vi "Add Canvas Wfm To Save.vi"(7 "Canvas Trim and Resample Settings":cluster{"Duration":dbl, "Sample Rate":dbl}={"Duration"=0.002, "Sample Rate"=0.0} {"Sample Rate" format="%#_6pHz"; "Duration" format="%#_6ps"}, 8 "error in (no error)":errorcluster, 9 "Canvas Wfm Array":waveform(dbl)[](array[waveform]), 10 "To Save Wfm Arrays In":waveform(dbl)[](array[waveform]), 11 "Channels Ctrl Ref":refnum<vi>) -> (0 "error out":errorcluster, 1 "Waveform Summary JSON":string[](array[string]), 2 "To Save Wfm Arrays Out":waveform(dbl)[](array[waveform]), 3 "Channel Names":string[](array[string]))   [LabVIEW 2025, in "TDMS Waveform Creator UI.lvlib"]
uses:
  TDMS Waveform Creator UI.lvlib
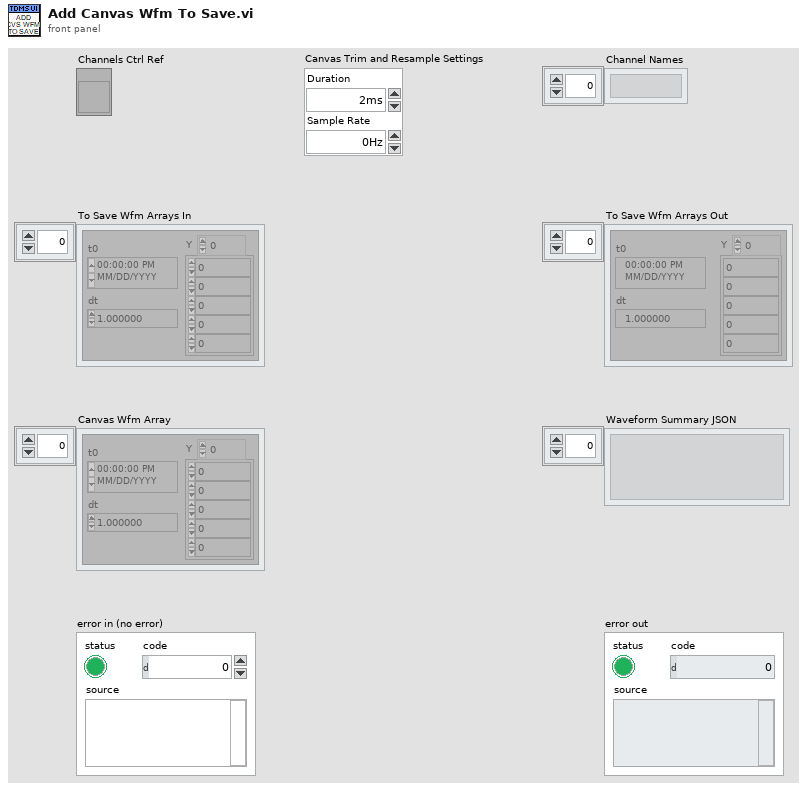
[diagram p1: front panel]
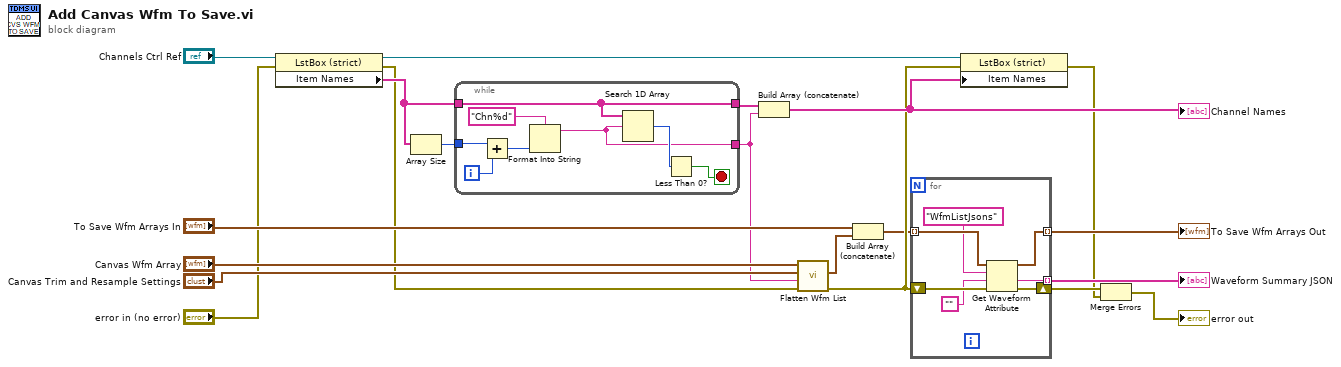
[diagram p0: block diagram]
diagram:
  n1 = property class="LstBox (strict)"(reference="Channels Ctrl Ref", error in="error in (no error)") -> (reference out=w8:refnum<vi>, error out=w2:errorcluster, "Item Names"=w9:string[])
  n2 = Array Size(array=w9) -> (size(s)=w11:i32)
  n3 = while {
    tunnel: w11 -> [w28]
    tunnel: w9 -> [w22]
    tunnel: [w23] -> w1
    tunnel: [w22] -> w10
    i -> [w26]
    stop <- w25 stop-if-true
    n4 = Add(x=w28, y=w26) -> (x+y=w27:i32)
    n5 = Format Into String(format string="Chn%d", w27) -> (resulting string=w23:string)  [unwired: 2 in, 1 out]
    n6 = Search 1D Array(1D array=w22, element=w23) -> (index of element=w24:i32)  [unwired: 1 in]
    n7 = Less Than 0?(x=w24) -> (x < 0?=w25:bool)
  }
  n8 = Build Array (concatenate)(w10, w1) -> (w14:string[])
  "Channel Names" <- w14
  n9 = call "Flatten Wfm List.vi"("error in (no error)"=w2, "Channel Name"=w1, "Trim and Resample Settings"="Canvas Trim and Resample Settings", "Canvas Wfm Array In"="Canvas Wfm Array") -> ("error out"=w7:errorcluster, "Final Flatten Wfm Channel"=w6:waveform(dbl))  [unwired: 5 in, 1 out]
  n10 = Build Array (concatenate)("To Save Wfm Arrays In", w6) -> (w4:waveform(dbl)[])
  n11 = for {
    shift-right: [w34] -> w5
    shift-left: w7 -> [w35]
    tunnel: w4 -> [w33] mode=indexing
    tunnel: [w32] -> w16 mode=indexing
    tunnel: [w29] -> w15 mode=indexing
    n12 = Get Waveform Attribute(4:w35, 5:"", 6:"WfmListJsons" ("name"), 7:w33) -> (0:w34:errorcluster, 1:w29:string, 3:w32:waveform(dbl))  [unwired: 1 out]
  }
  "To Save Wfm Arrays Out" <- w16
  "Waveform Summary JSON" <- w15
  n13 = property class="LstBox (strict)"(reference=w8, error in=w7, "Item Names"=w14) -> (error out=w3:errorcluster)  [unwired: 1 out]
  n14 = Merge Errors(w5, w3) -> (→"error out":errorcluster)
